vi "Read_SPI-4xUart (SubVI).vi"(0 "Number of Bytes to read (Hex)":u32, 5 "Channel Name":tag="A/SPI", 7 "SPI User Configuration":T1={"Frequency [Hz]"=400000.0, "Clock Phase"=enum."Leading", "Clock Polarity"=enum."Low", "Data Direction"=enum."Least significant bit first", "Frame Length"=8} {"Frame Length" min=1 max=16}, 11 "error in (no error)":errorcluster) -> (4 "Data Received":u16[](array[numeric]), 15 "error out":errorcluster)   [LabVIEW 2018]
uses:
  <vilib>/myRIO/Instrument Drivers/Onboard IO/SPI/SPI.lvlib
  <vilib>/myRIO/Common/Instrument Driver Framework/myRIO v1.0/SPI/typedefs/SPI Clock Phase.ctl
  <vilib>/myRIO/Common/Instrument Driver Framework/myRIO v1.0/SPI/typedefs/SPI Clock Polarity.ctl
  <vilib>/myRIO/Common/Instrument Driver Framework/myRIO v1.0/SPI/typedefs/SPI Data Direction.ctl
  <vilib>/myRIO/Common/Instrument Driver Framework/myRIO v1.0/SPI/typedefs/SPI Frame Length.ctl
  <vilib>/myRIO/Instrument Drivers/Onboard IO/SPI/typedefs/SPI User Configuration.ctl
panel:
  out "Data String":string
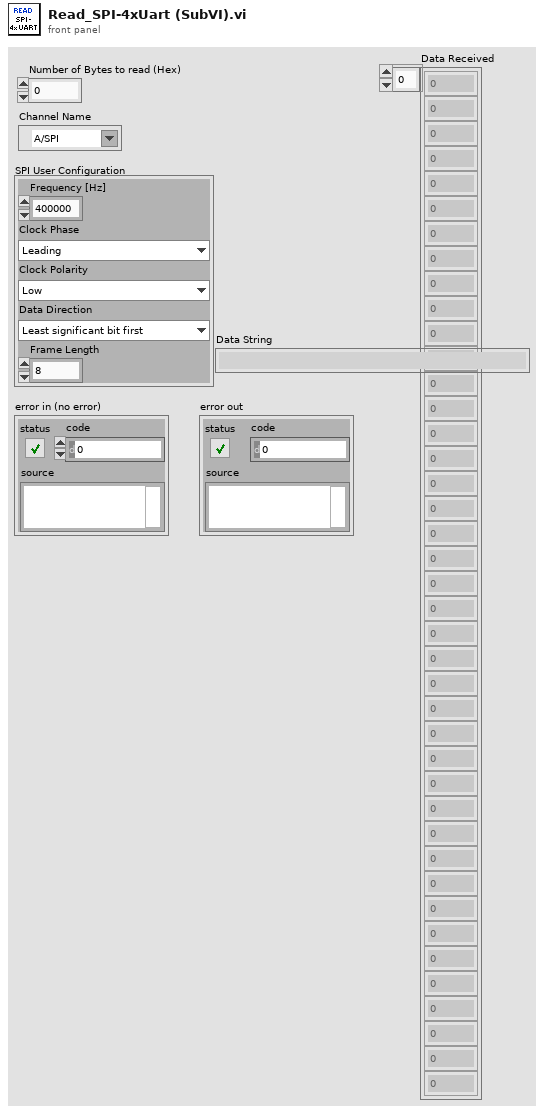
[diagram p1: front panel]
types:
  T1 = typedef "SPI.lvlib/SPI User Configuration.ctl" = cluster{"Frequency [Hz]":dbl, "Clock Phase":T2, "Clock Polarity":T3, "Data Direction":T4, "Frame Length":T5}
  T2 = typedef "SPI Clock Phase.ctl" = enum8{"Leading", "Trailing"}
  T3 = typedef "SPI Clock Polarity.ctl" = enum8{"Low", "High"}
  T4 = typedef "SPI Data Direction.ctl" = enum8{"Most significant bit first", "Least significant bit first"}
  T5 = typedef "SPI Frame Length.ctl" = u8
  T6 = typedef "SPI.lvlib/SPI Reference.ctl" = cluster{"myRIO Reference":T7, "SPI Channels Enum":T11, "SPI Configuration":T12}
  T7 = typedef "myRIO Generic Hardware Reference.ctl" = cluster{"myRIO Model":T8, "myRIO Hardware Reference":T9}
  T8 = typedef "Hardware Version Enum.ctl" = enum16{"Unknown", "myRIO-1900", "myRIO-1950", "roboRIO", "NI ELVIS RIO CM", "ELVIS III"}
  T9 = typedef "myRIO v1.0 Reference.ctl" = cluster{"Generic FPGA Reference":T10, "Allow multiple opens":bool}
  T10 = typedef "Generic FPGA Reference.ctl" = refnum<k20>
  T11 = typedef "SPI Channels Enum.ctl" = enum16{"Not Connected", "A/SPI", "B/SPI", "SPI/SPI"}
  T12 = typedef "SPI.lvlib/SPI Configuration.ctl" = cluster{"Frequency [Hz]":dbl, "Clock Phase":T2, "Clock Polarity":T3, "Data Direction":T4, "Frame Length":T5}
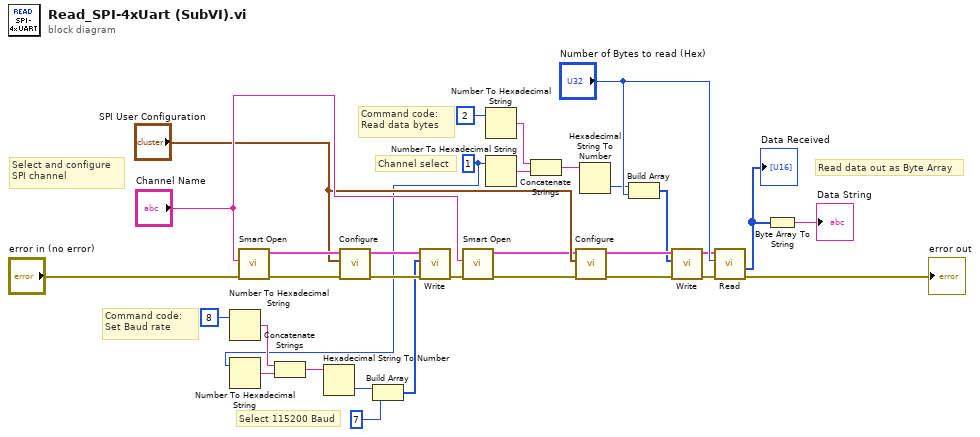
[diagram p0: block diagram]
diagram:
  w1 = 1 ("number")
  # "Read data out as Byte Array"
  # "Select and configure \nSPI channel"
  # "Select 115200 Baud"
  # "Command code: \nSet Baud rate"
  # "Channel select"
  # "Command code: \nRead data bytes"
  n1 = Number To Hexadecimal String(2:8 ("number")) -> (0:w8:string)  [unwired: 1 in]
  n2 = Number To Hexadecimal String(2:w1) -> (0:w7:string)  [unwired: 1 in]
  n3 = call <vilib>:"Smart Open.vi"("error in (no error)"="error in (no error)", "Channel Name"="Channel Name") -> ("error out"=w30:errorcluster, "SPI Ref Out"=w29:T6)  [unwired: 8 in]
  n4 = Concatenate Strings(w8, w7) -> (w6:string)
  n5 = Hexadecimal String To Number(string=w6) -> (number=w5:u32)  [unwired: 2 in, 1 out]
  n6 = call <vilib>:"Configure.vi"("error in (no error)"=w30, "SPI User Configuration"="SPI User Configuration", "SPI Ref In"=w29) -> ("error out"=w27:errorcluster, "SPI Ref Out"=w28:T6)  [unwired: 7 in]
  n7 = Build Array(w5, u32 7 ("element")) -> (w3:u32[])
  n8 = call <vilib>:"Write.vi"("error in (no error)"=w27, "Frames to Write"=w3, "SPI Ref In"=w28) -> ("error out"=w26:errorcluster)  [unwired: 7 in, 1 out]
  n9 = call <vilib>:"Smart Open.vi"("error in (no error)"=w26, "Channel Name"="Channel Name") -> ("error out"=w16:errorcluster, "SPI Ref Out"=w15:T6)  [unwired: 8 in]
  n10 = Number To Hexadecimal String(2:2 ("number")) -> (0:w21:string)  [unwired: 1 in]
  n11 = Number To Hexadecimal String(2:w1) -> (0:w20:string)  [unwired: 1 in]
  n12 = Concatenate Strings(w21, w20) -> (w19:string)
  n13 = call <vilib>:"Configure.vi"("error in (no error)"=w16, "SPI User Configuration"="SPI User Configuration", "SPI Ref In"=w15) -> ("error out"=w12:errorcluster, "SPI Ref Out"=w13:T6)  [unwired: 7 in]
  n14 = Hexadecimal String To Number(string=w19) -> (number=w18:u32)  [unwired: 2 in, 1 out]
  n15 = Build Array(w18, "Number of Bytes to read (Hex)") -> (w11:u32[])
  n16 = call <vilib>:"Write.vi"("error in (no error)"=w12, "Frames to Write"=w11, "SPI Ref In"=w13) -> ("error out"=w10:errorcluster, "SPI Ref Out"=w9:T6)  [unwired: 7 in]
  n17 = call <vilib>:"Read.vi"("error in (no error)"=w10, "Frame Count"="Number of Bytes to read (Hex)", "SPI Ref In"=w9) -> ("error out"=→"error out":errorcluster, "Frames Read"=w22:u16[])  [unwired: 5 in, 1 out]
  "Data Received" <- w22
  n18 = Byte Array To String(unsigned byte array=w22) -> (string=→"Data String":string)
